vi "light_center_finder.vi"(4 "Home pose":dbl[](array[numeric])=[0.25469575119784055, -16.45995133588347, 3.732397870471535, 0.0, 0.0, 0.0] format="%#.3f", 5 "Stage orientation":T1 format="%#_3f", 6 "Half angle (degrees)":dbl=10.0, 7 "Pivot point":dbl[](array[numeric])=[0.0, 0.0, 0.0, 0.0, 0.0, 0.0], 9 "Point selector":T3={"Pose mode"=enum."Light", "Light number"=5} {"Light number" min=0 max=5}, 10 "Axis":i32, 11 "Override":T2) -> (1 "Light offset (stage coords)":dbl[](array[numeric]) format="%#_4g", 2 "magnitude":dbl, 3 "Off axis":dbl)   [LabVIEW 2013]
uses:
  calibration/point_selector.ctl
  ui_override_opts.ctl
  <vilib>/Analysis/Matrix/Datatypes/RealMatrix.ctl
  <vilib>/Analysis/baseanly.llb/A x Vector.vi
  utilities/labview/norm_vec.vi
  <vilib>/Analysis/NI_AALBase.lvlib
  <vilib>/Analysis/Matrix/NI_Matrix.lvlib
panel:
  # "Do one axis sweep to locate light position."
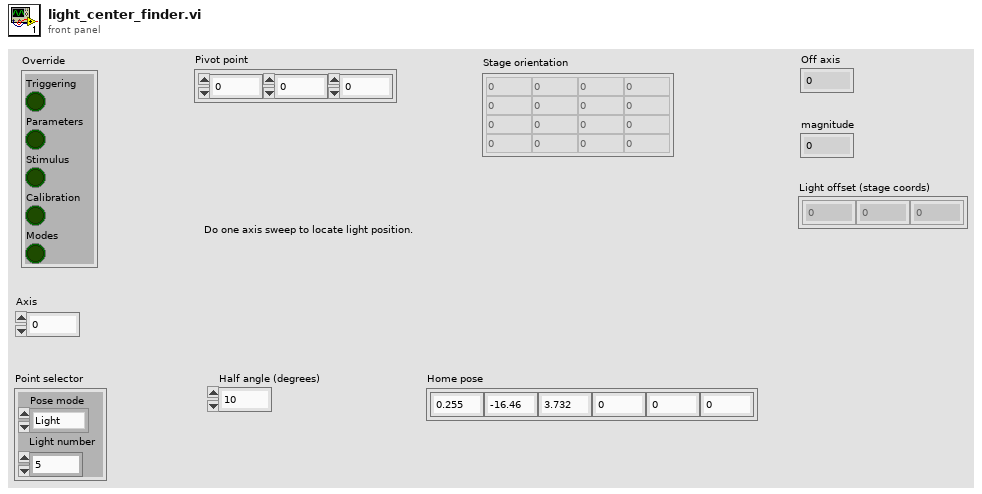
[diagram p1: front panel]
types:
  T1 = typedef "NI_Matrix.lvlib/RealMatrix.ctl" = dbl[][]
  T2 = typedef "ui_override_opts.ctl" = cluster{"Triggering":bool, "Parameters":bool, "Stimulus":bool, "Calibration":bool, "Modes":bool}
  T3 = typedef "point_selector.ctl" = cluster{"Pose mode":enum16{"Light", "Handle", "Output"}, "Light number":i32}
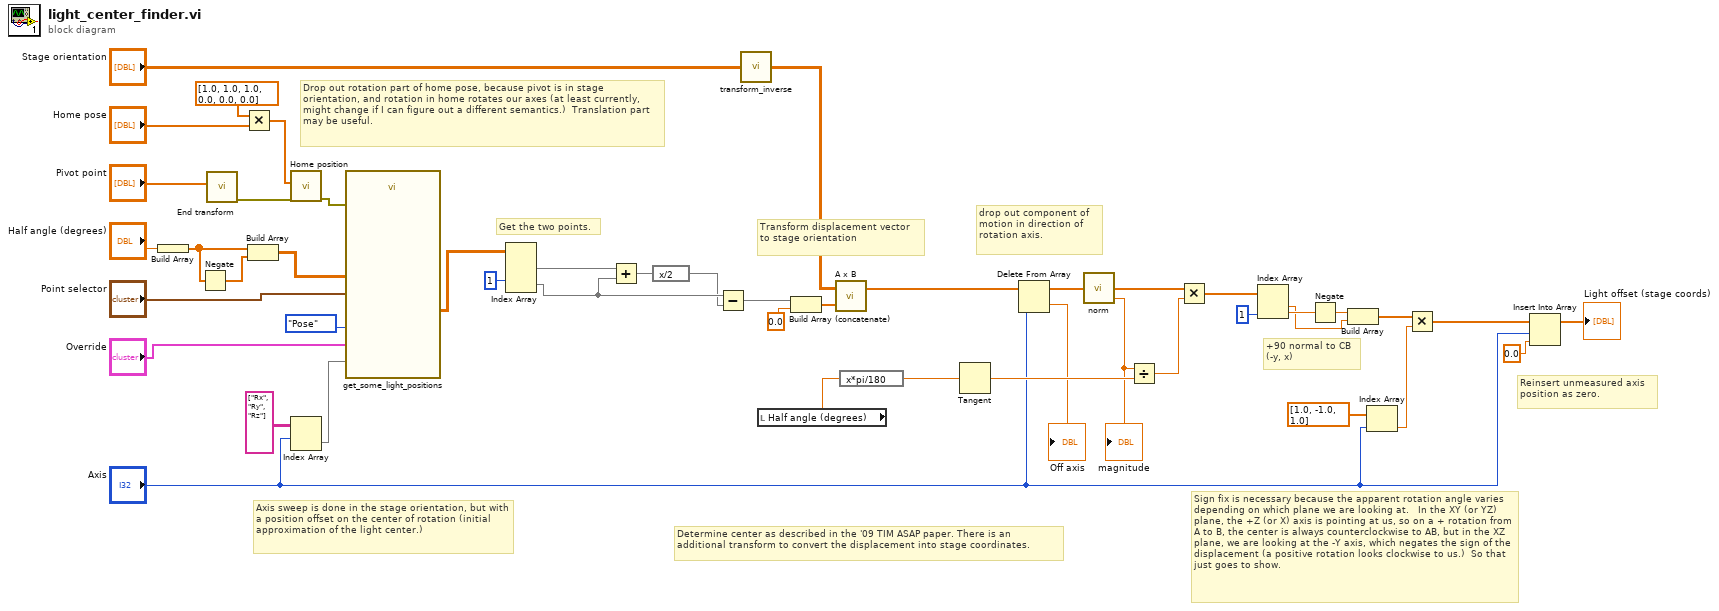
[diagram p0: block diagram]
diagram:
  # "Drop out rotation part of home pose, because pivot is in stage orientation, and rotation in home rotates our axes (at least currently, might change if I can figure out a different semantics.)  Translation part may be useful."
  # "Sign fix is necessary because the apparent rotation angle varies depending on which plane we are looking at.   In the XY (or YZ) plane, the +Z (or X) axis is pointing at us, so on a + rotation from A to B, the center is always counterclockwise to AB, but in the XZ plane, we are looking at the -Y axis, which negates the sign of the displacement (a positive rotation looks clockwise to us.)  So that just goes to show."
  # "Determine center as described in the '09 TIM ASAP paper. There is an additional transform to convert the displacement into stage coordinates."
  # "Reinsert unmeasured axis position as zero."
  # "Axis sweep is done in the stage orientation, but with a position offset on the center of rotation (initial approximation of the light center.)"
  # "Transform displacement vector to stage orientation"
  # "+90 normal to CB\n(-y, x)"
  # "drop out component of motion in direction of rotation axis."
  # "Get the two points."
  n1 = Build Array("Half angle (degrees)") -> (w42:dbl[])
  n2 = Negate(x=w42) -> (-x=w41:dbl[])
  n3 = call "End transform.vi"("End transform"="Pivot point") -> ("error out"=w17:errorcluster)  [unwired: 10 in]
  n4 = Multiply(x=dbl[] [1.0, 1.0, 1.0, 0.0, 0.0, 0.0], y="Home pose") -> (x*y=w2:dbl[])
  n5 = Build Array(w42, w41) -> (w40:dbl[][])
  n6 = call "Home position.vi"("error in"=w17, "Home position"=w2) -> ("error out"=w16:errorcluster)  [unwired: 9 in]
  n7 = Index Array(array=string[][] [["Rx"], ["Ry"], ["Rz"]] ("Axis names"), index (row)="Axis") -> (element=w38:string[])  [unwired: 1 in]
  n8 = call "get_some_light_positions.vi"("Point selector"="Point selector", "Position mode"=enum16{"Absolute axis", "Relative axis", "Pose"}."Pose", "error in"=w16, "Sequence"=w40, "Axis names"=w38, "Override"="Override") -> ("Light positions"=w8:sgl[][])  [unwired: 3 in, 2 out]
  n9 = Index Array(array=w8, index (row) #2=1 ("index (row)")) -> (element #1=w47:sgl[], element #2=w46:sgl[])  [unwired: 3 in]
  n10 = Add(x=w47, y=w46) -> (x+y=w35:sgl[])
  n11 = expression code="x/2"(w35) -> (w25:sgl[])
  n12 = Subtract(x=w46, y=w25) -> (x-y=w7:sgl[])
  n13 = call "transform_inverse.vi"("Transform"="Stage orientation") -> ("Inverse transform"=w9:T1)
  n14 = local read "Half angle (degrees)"() -> (w24:dbl)
  n15 = Build Array (concatenate)(w7, sgl 0.0) -> (w5:sgl[])
  n16 = call-poly <vilib>:"A x B.vi"("Vector"=w5, "A"=w9) -> ("A x Vector"=w6:dbl[])  [unwired: 1 out]
  n17 = expression code="x*pi/180"(w24) -> (w34:dbl)
  n18 = Tangent(1:w34) -> (0:w33:dbl)
  n19 = Delete From Array(array=w6, index="Axis") -> (deleted portion=→"Off axis":dbl, array with subset deleted=w30:dbl[])  [unwired: 1 in]
  n20 = call-poly "norm.vi"("vector"=w30) -> ("magnitude"=w23:dbl, "normalized vector"=w32:dbl[])  [unwired: 3 in]
  "magnitude" <- w23
  n21 = Divide(x=w23, y=w33) -> (x/y=w31:dbl)
  n22 = Multiply ("Multiply.vi")(x=w32, y=w31) -> (x*y=w15:dbl[])
  n23 = Index Array(array=w15, index #2=1 ("index")) -> (element #1=w26:dbl, element #2=w27:dbl)  [unwired: 1 in]
  n24 = Negate(x=w27) -> (-x=w28:dbl)
  n25 = Build Array(w28, w26) -> (w14:dbl[])
  n26 = Index Array(array=dbl[] [1.0, -1.0, 1.0], index="Axis") -> (element=w11:dbl)
  n27 = Multiply(x=w14, y=w11) -> (x*y=w13:dbl[])
  n28 = Insert Into Array(array=w13, index="Axis", new element=0.0 ("new element/subarray")) -> (→"Light offset (stage coords)":dbl[])
